vi "Check_Pos_L.vi"(0 "FPGA_Data":sgl[](array[numeric]), 2 "Q_MotorCmd_IN":refnum<queue>, 3 "Q_MotorCmd_Err_IN":errorcluster, 7 "Param_In":T1) -> (6 "LOAD_CELL_PEAK_L":sgl[](array[numeric]), 12 "Target_Pos":i32, 13 "Param_Out":T1, 14 "Flag":T2(ring), 15 "L_NUM":u32, 16 "Q_MotorCmd_OUT":refnum<queue>, 17 "Q_MotorCmd_Err_OUT":errorcluster, 18 "L_Period":u32, 19 "L_GCP":sgl)   [LabVIEW 2019]
uses:
  RT_GLOBAL.vi
panel:
  out "L_Period_EXT":u32
  out "L_GCP_EXT":sgl
  out "L_NUM_EXT":u32
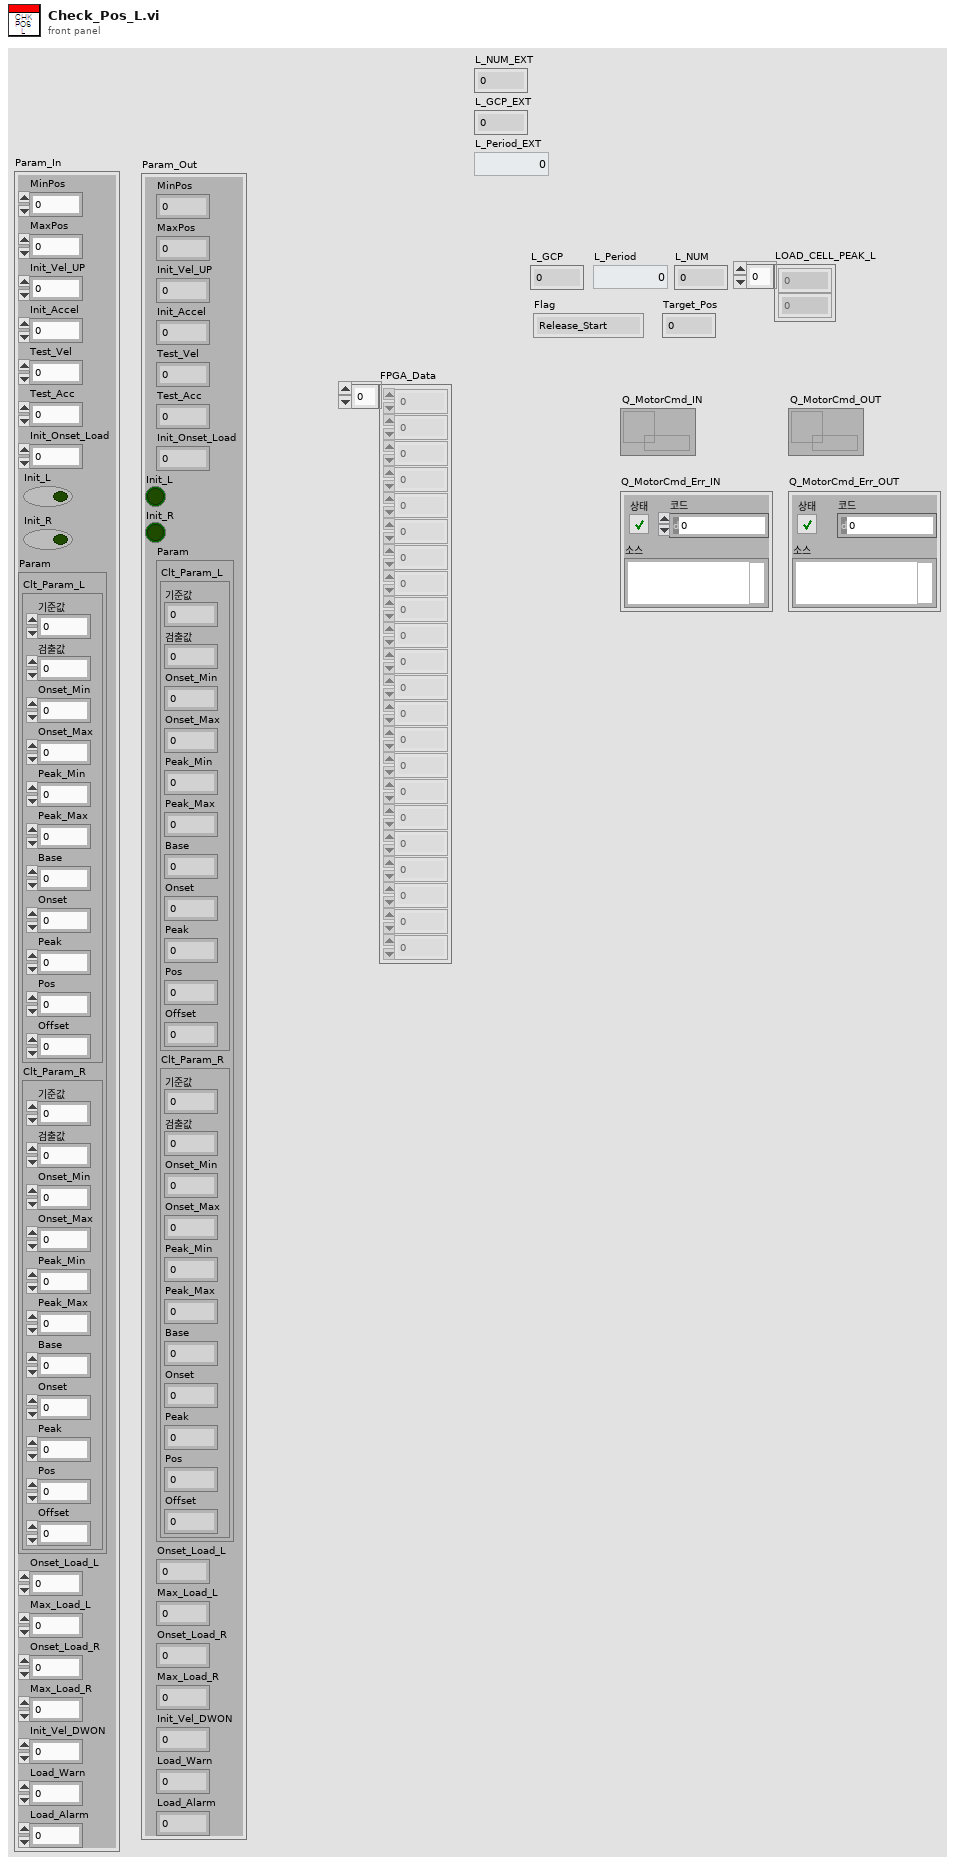
[diagram p1: front panel]
types:
  T1 = cluster{"MinPos":i32, "MaxPos":i32, "Init_Vel_UP":i32, "Init_Accel":u32, "Test_Vel":i32, "Test_Acc":u32, "Init_Onset_Load":sgl, "Init_L":bool, "Init_R":bool, "Param":cluster{"Clt_Param_L":cluster{"기준값":sgl, "검출값":sgl, "Onset_Min":sgl, "Onset_Max":sgl, "Peak_Min":sgl, "Peak_Max":sgl, "Base":i32, "Onset":i32, "Peak":i32, "Pos":i32, "Offset":sgl}, "Clt_Param_R":cluster{"기준값":sgl, "검출값":sgl, "Onset_Min":sgl, "Onset_Max":sgl, "Peak_Min":sgl, "Peak_Max":sgl, "Base":i32, "Onset":i32, "Peak":i32, "Pos":i32, "Offset":sgl}}, "Onset_Load_L":sgl, "Max_Load_L":sgl, "Onset_Load_R":sgl, "Max_Load_R":sgl, "Init_Vel_DWON":i32, "Load_Warn":sgl, "Load_Alarm":sgl}
  T2 = enum16{"Release_Start", "Onset_Start", "Peak_Start", "Calculate"}
  T3 = cluster{"Cmd":string, "Data1":variant, "Data2":variant}
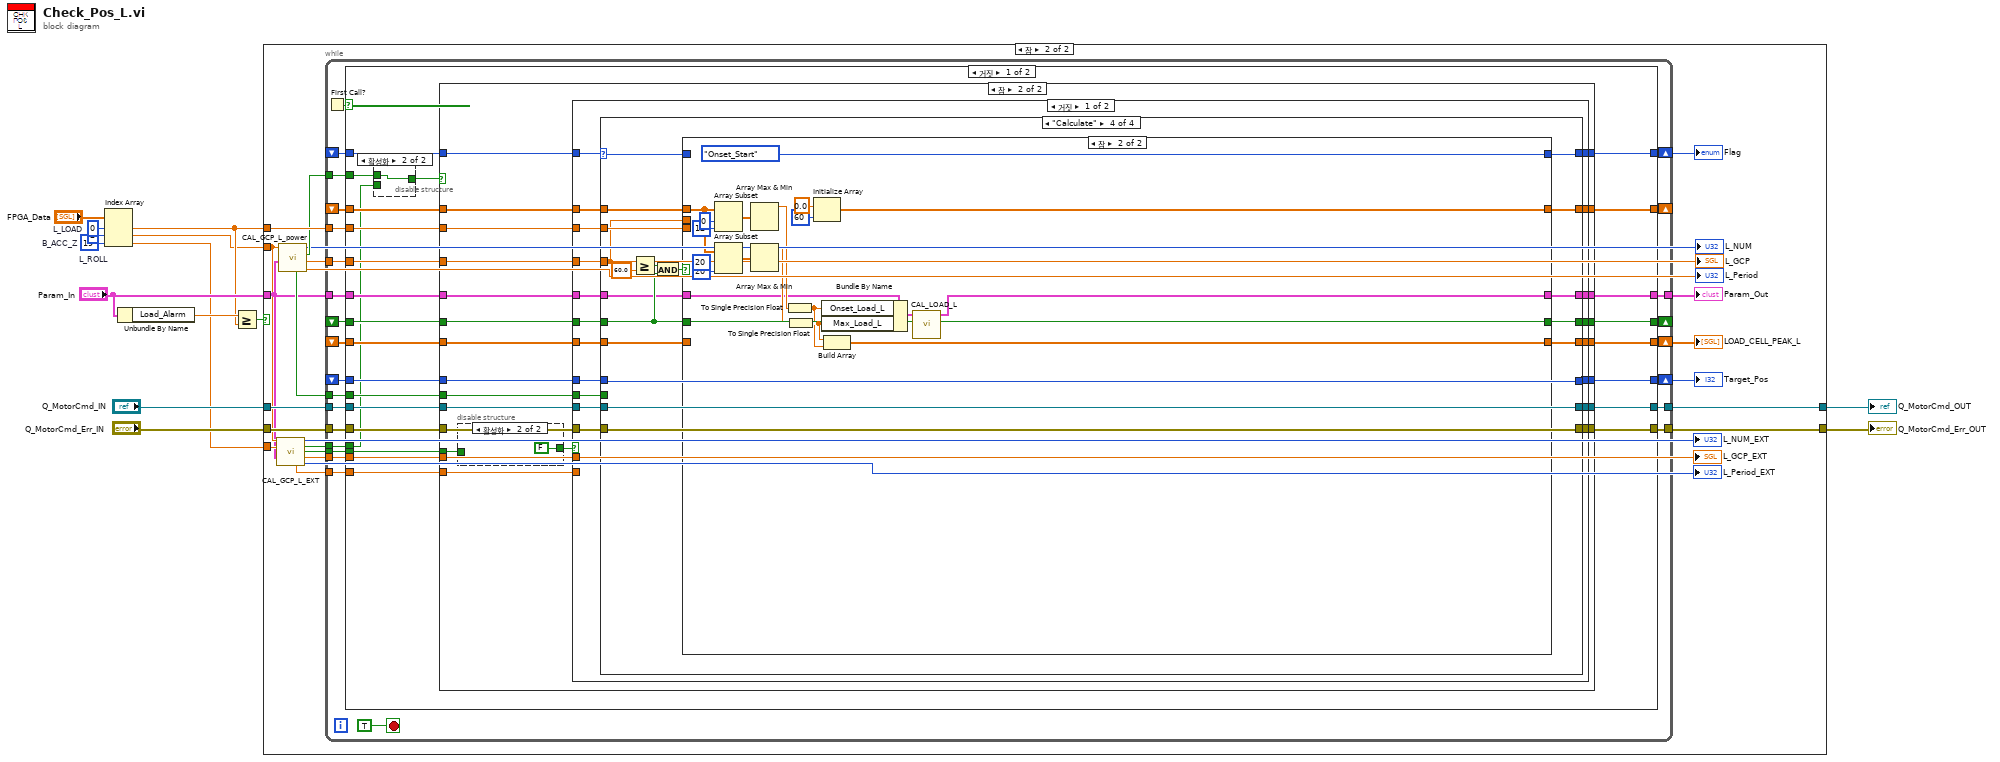
[diagram p0: block diagram]
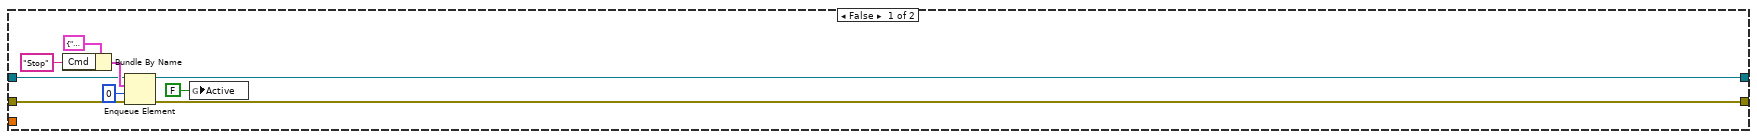
[diagram p2: hidden frame]
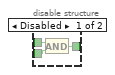
[diagram p3: hidden frame]
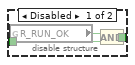
[diagram p5: hidden frame]
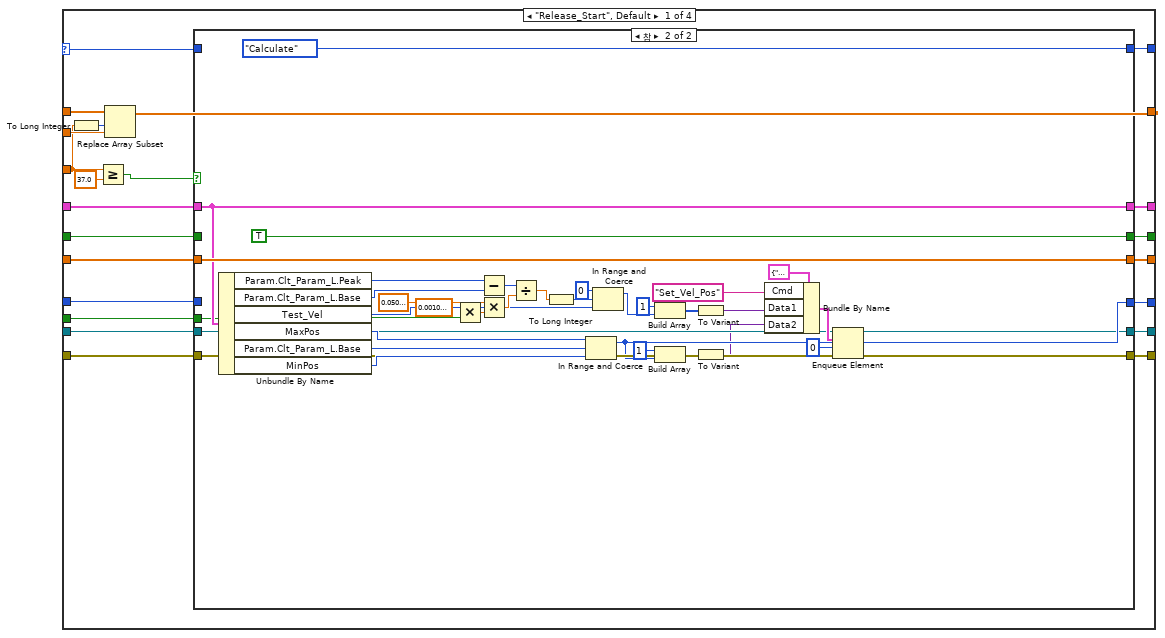
[diagram p6: hidden frame]
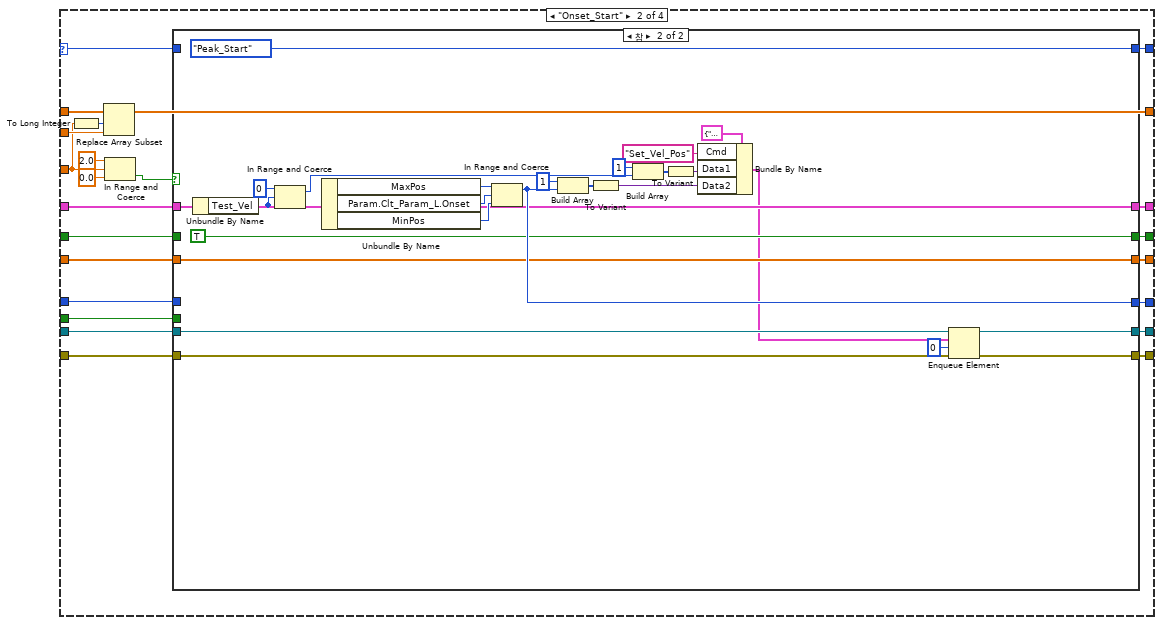
[diagram p8: hidden frame]
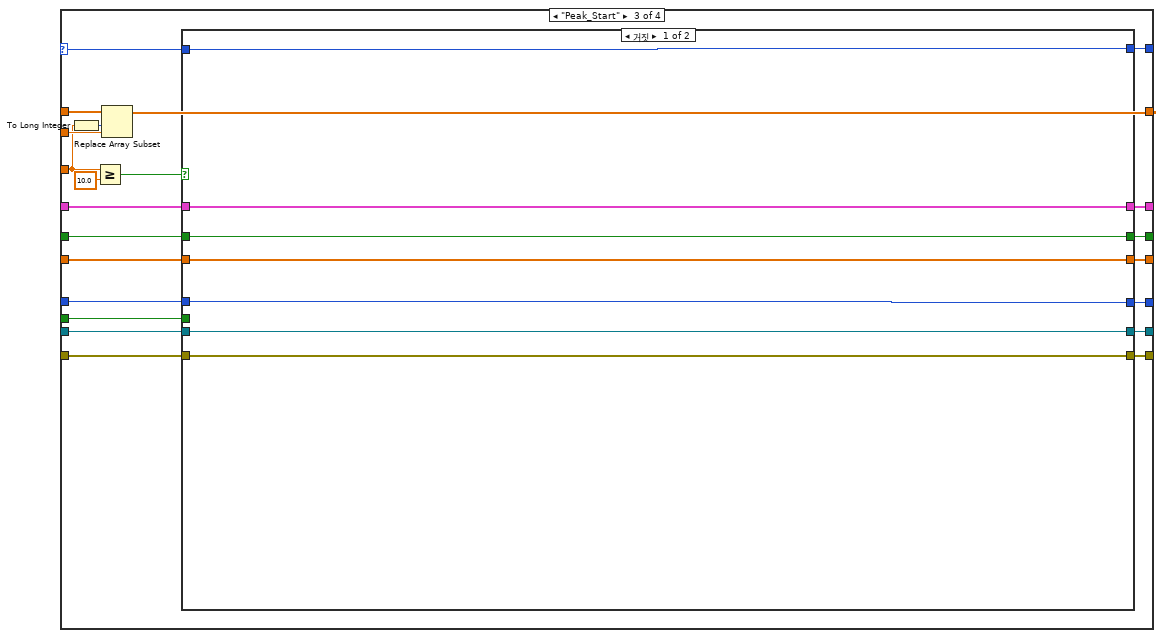
[diagram p10: hidden frame]
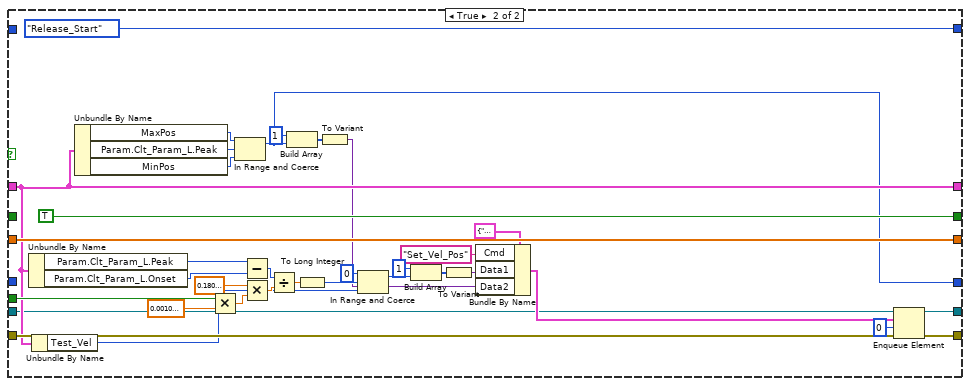
[diagram p11: hidden frame]
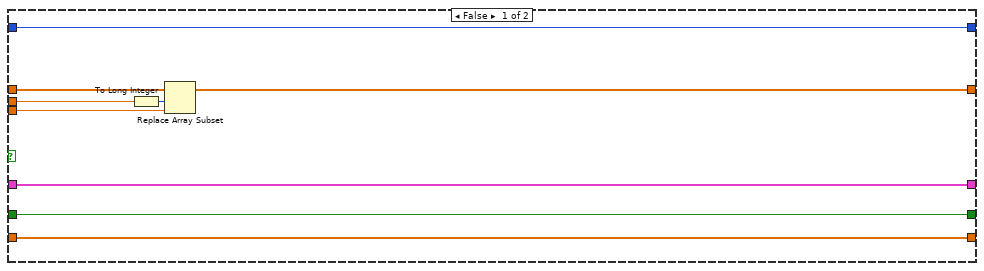
[diagram p12: hidden frame]
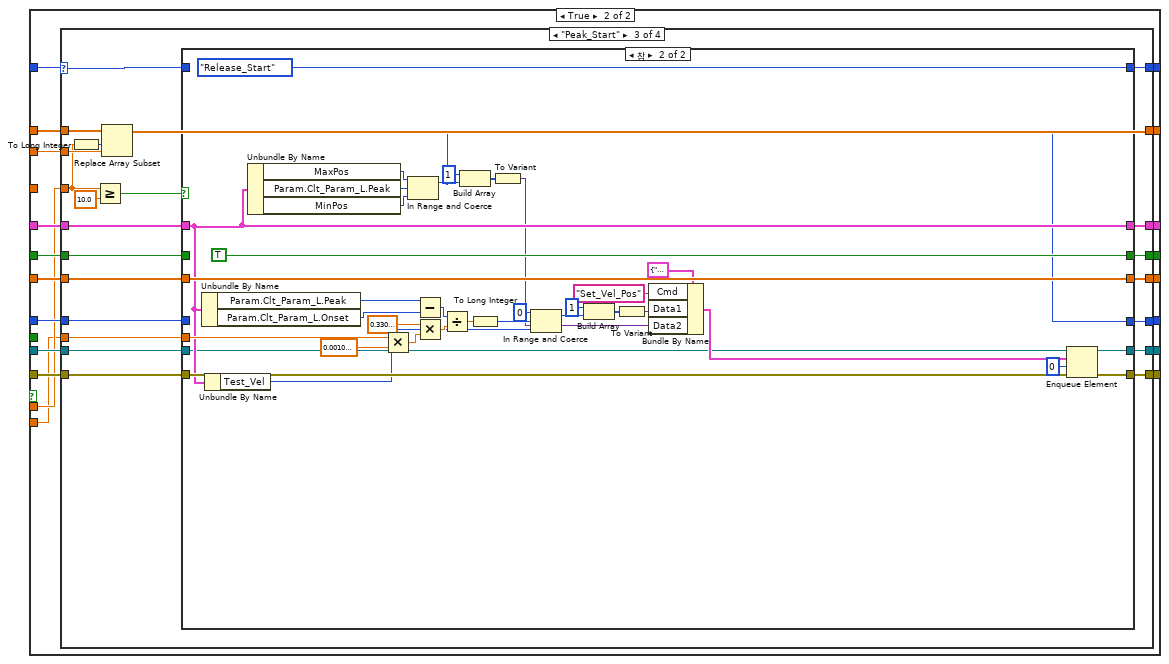
[diagram p13: hidden frame]
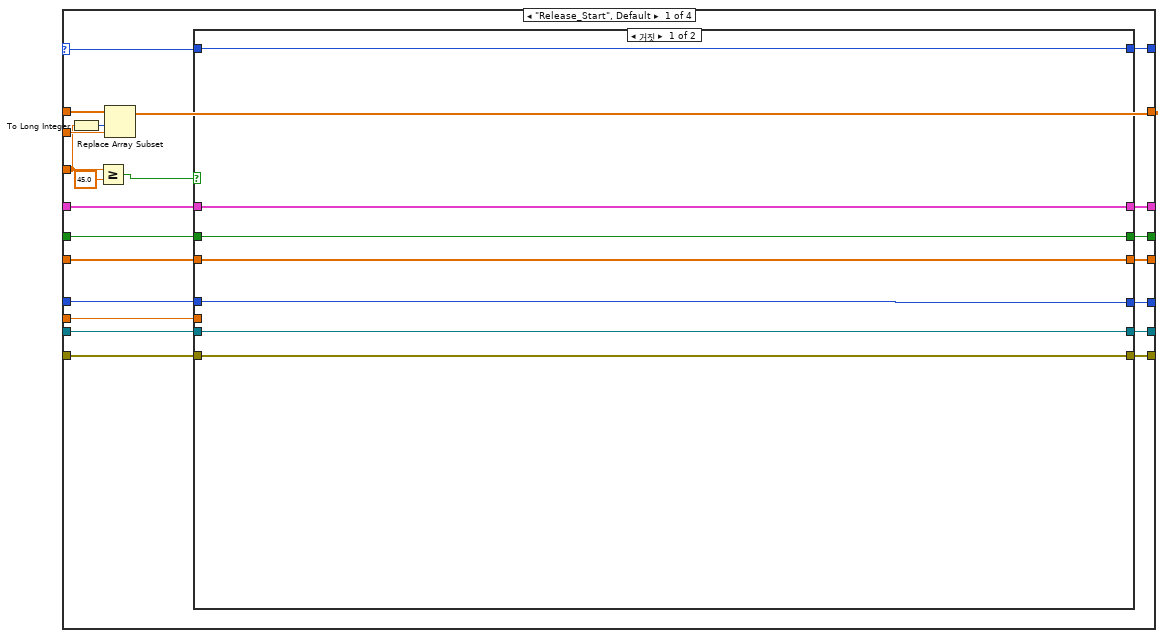
[diagram p14: hidden frame]
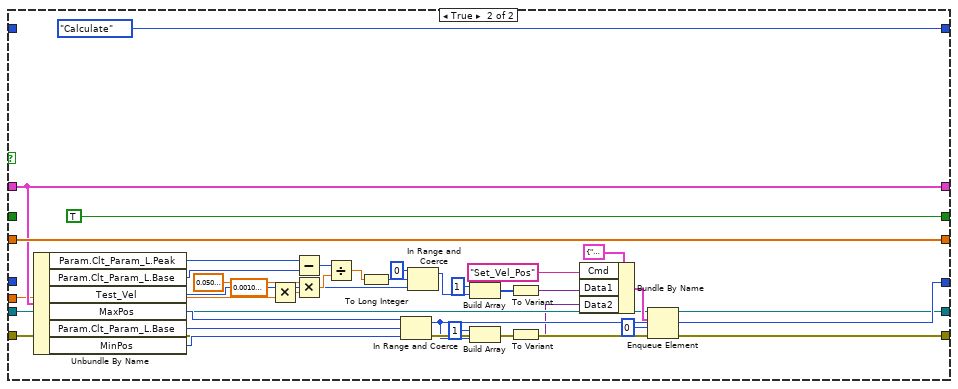
[diagram p15: hidden frame]
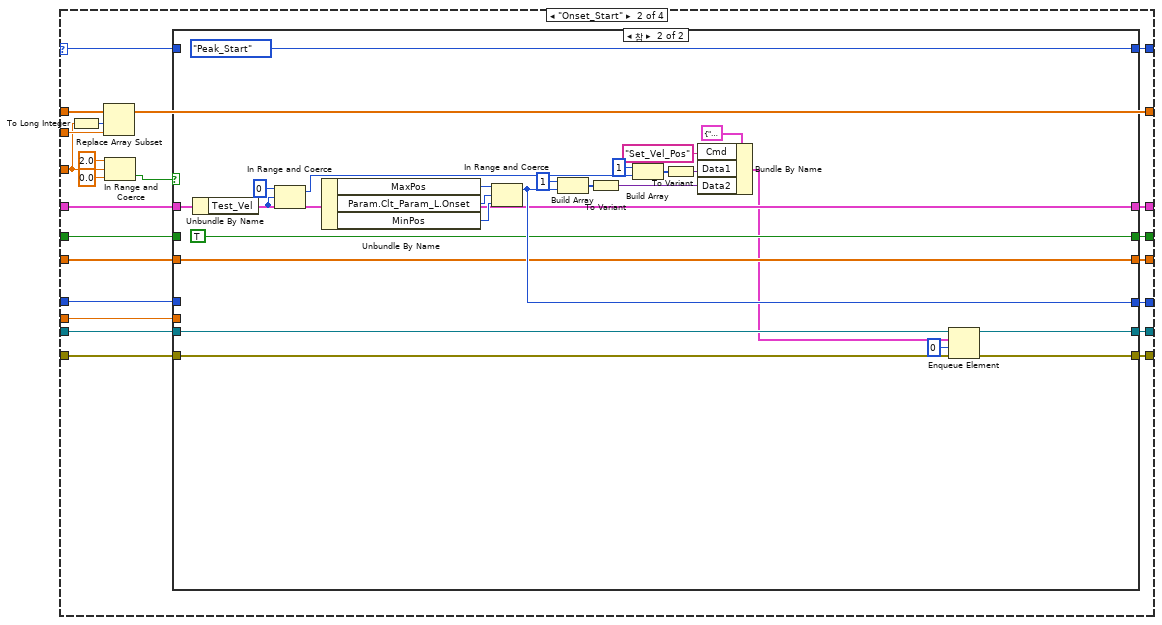
[diagram p16: hidden frame]
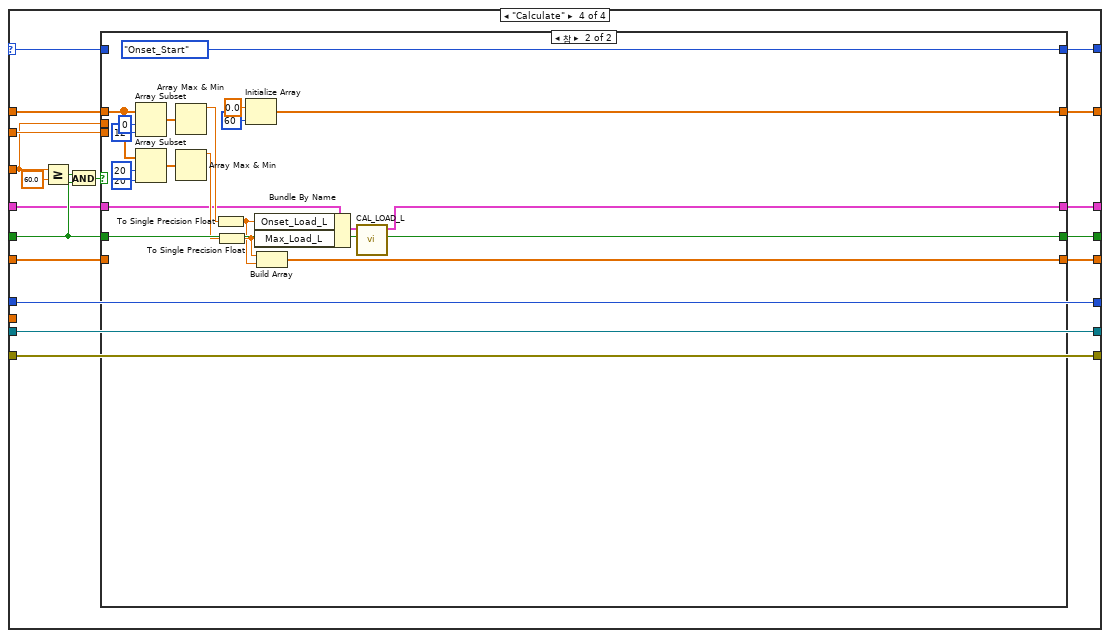
[diagram p19: hidden frame]
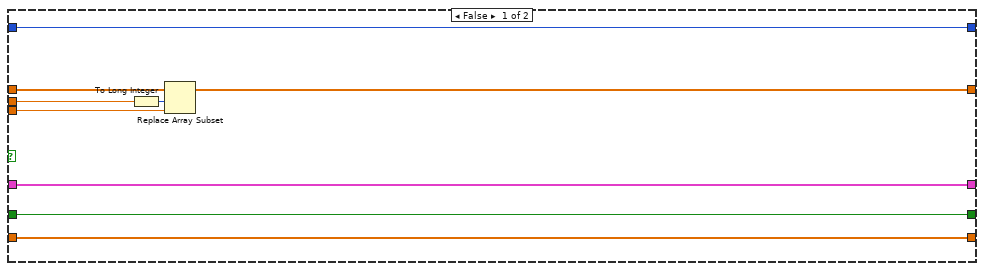
[diagram p20: hidden frame]
diagram:
  w4 = 19  # B_ACC_Z
  w6 = 2  # L_ROLL
  w8 = 0  # L_LOAD
  n1 = Index Array(array="FPGA_Data", index #1=w8, index #2=w6, index #3=w4) -> (element #1=w7:sgl, element #2=w5:sgl, element #3=w3:sgl)
  n2 = Unbundle By Name("Param_In") -> ("Load_Alarm"=w12:sgl)
  n3 = Greater Or Equal?(x=w12, y=w7) -> (x >= y?=w11:bool)
  n4 = case shown="참" w11 {
    tunnel: w5 -> [_ w34]
    tunnel: "Q_MotorCmd_IN" -> [w20 w46]
    tunnel: "Q_MotorCmd_Err_IN" -> [w19 w45]
    tunnel: "Param_In" -> [_ w32]
    tunnel: w7 -> [_ w44]
    tunnel: w3 -> [_ w33]
    tunnel: [w16 w25] -> w2
    tunnel: [w15 w24] -> w1
    frame False {
      n5 = Bundle By Name(cluster=T3 {"Cmd"="", "Data1"=variant, "Data2"=variant}, "Cmd"="Stop") -> (w21:T3)
      n6 = Enqueue Element(queue=w20, element=w21, timeout in ms (-1)=0 ("타임아웃(ms) (-1)"), error in (no error)=w19) -> (queue out=w16:refnum<queue>, error out=w15:errorcluster)  [unwired: 1 out]
      n7 = global write "RT_GLOBAL.vi" "Active"(FALSE ("Active")) -> ()
    }
    frame True {
      n8 = call "CAL_GCP_L_EXT.vi"("L_ROLL"=w34, "ACC_Z"=w33, "Param_In"=w32) -> ("L_NUM"=→"L_NUM_EXT":u32, "L_Ctrl_Start"=w29:bool, "L_RUN_OK"=w28:bool, "L_GCP_EXT"=w27:sgl, "L_GCP_Total_TIME"=w26:sgl, "L_Period"=→"L_Period_EXT":u32)  [unwired: 7 in]
      "L_GCP_EXT" <- w27
      n9 = call "CAL_GCP_L_power.vi"("출력 클러스터 2"=w32, "L_ROLL"=w34) -> ("L_Period"=→"L_Period":sgl, "L_GCP"=w42:sgl, "L_Ctrl_Start"=w43:bool, "L_NUM"=→"L_NUM":u32, "L_Run_OK"=w35:bool)  [unwired: 5 in]
      "L_GCP" <- w42
      n10 = while {
        tunnel: w43 -> [w70]
        tunnel: w42 -> [w56]
        shift-right: [w71] -> w39
        shift-left: _ -> [w62]
        shift-right: [w69] -> _
        shift-left: _ -> [w61]
        tunnel: w32 -> [w68]
        tunnel: [w67] -> w36
        shift-right: [w65] -> _
        shift-left: _ -> [w66]
        shift-right: [w64] -> w38
        shift-left: _ -> [w59]
        tunnel: w46 -> [w58]
        tunnel: w45 -> [w57]
        tunnel: w44 -> [w60]
        shift-right: [w55] -> w37
        shift-left: _ -> [w54]
        tunnel: w35 -> [w53]
        tunnel: w29 -> [w52]
        tunnel: w28 -> [w51]
        tunnel: w27 -> [w50]
        tunnel: w26 -> [w49]
        tunnel: [w48] -> w25
        tunnel: [w47] -> w24
        stop <- TRUE stop-if-true
        n11 = First Call?() -> (First Call?: T/F=w72:bool)
        n12 = case shown="거짓" w72 {
          tunnel: [w97 T2."Release_Start"] -> w71
          tunnel: w70 -> [w80 _]
          tunnel: [w94 w642] -> w69
          tunnel: [w91 w641] -> w67
          tunnel: w68 -> [w92 w641]
          tunnel: w66 -> [w89 _]
          tunnel: [w90 TRUE] -> w65
          tunnel: [w87 0] -> w64
          tunnel: w62 -> [w96 _]
          tunnel: w61 -> [w95 _]
          tunnel: w60 -> [w93 _]
          tunnel: w59 -> [w88 _]
          tunnel: w58 -> [w86 w636]
          tunnel: w57 -> [w85 w635]
          tunnel: w56 -> [w84 _]
          tunnel: [w83 w637] -> w55
          tunnel: w54 -> [w82 _]
          tunnel: w53 -> [w81 _]
          tunnel: w52 -> [w79 _]
          tunnel: w51 -> [w77 _]
          tunnel: w50 -> [w76 _]
          tunnel: w49 -> [w75 _]
          tunnel: [w74 w636] -> w48
          tunnel: [w73 w635] -> w47
          frame False {
            n13 = disable-structure shown="활성화" {
              disable-tunnel: w80 -> [w100 w101]
              disable-tunnel: w79 -> [w99 _]
              disable-tunnel: [w98 w101] -> w78
              frame Disabled {
                n14 = And(x=w100, y=w99) -> (x .and. y?=w98:bool)
              }
              frame Enabled {
              }
            }
            n15 = case shown="참" w78 {
              tunnel: [w109 w131] -> w97
              tunnel: w96 -> [w109 w132]
              tunnel: [w108 w129] -> w94
              tunnel: w95 -> [w108 w130]
              tunnel: w93 -> [_ w127]
              tunnel: [w107 w125] -> w91
              tunnel: w92 -> [w107 w126]
              tunnel: [w106 w124] -> w90
              tunnel: w89 -> [w106 w123]
              tunnel: [w105 w122] -> w87
              tunnel: w88 -> [w105 w121]
              tunnel: w86 -> [w103 w120]
              tunnel: w85 -> [w102 w119]
              tunnel: w84 -> [_ w128]
              tunnel: [w104 w118] -> w83
              tunnel: w82 -> [w104 w117]
              tunnel: w81 -> [_ w116]
              tunnel: w77 -> [_ w113]
              tunnel: w76 -> [_ w114]
              tunnel: w75 -> [_ w112]
              tunnel: [w103 w111] -> w74
              tunnel: [w102 w110] -> w73
              frame False {
              }
              frame True {
                n16 = disable-structure shown="활성화" {
                  disable-tunnel: [w135 FALSE] -> w115
                  disable-tunnel: w113 -> [w134 _]
                  frame Disabled {
                    n17 = global read "RT_GLOBAL.vi" "R_RUN_OK"() -> (w133:bool)
                    n18 = And(x=w133, y=w134) -> (x .and. y?=w135:bool)
                  }
                  frame Enabled {
                  }
                }
                n19 = case shown="거짓" w115 {
                  tunnel: w132 -> [w155 w404]
                  tunnel: [w154 w403] -> w131
                  tunnel: w130 -> [w153 w402]
                  tunnel: [w152 w401] -> w129
                  tunnel: w128 -> [w151 _]
                  tunnel: w127 -> [w150 w400]
                  tunnel: w126 -> [w149 w399]
                  tunnel: [w148 w398] -> w125
                  tunnel: [w147 w397] -> w124
                  tunnel: w123 -> [w146 w396]
                  tunnel: [w145 w395] -> w122
                  tunnel: w121 -> [w144 w394]
                  tunnel: w120 -> [w143 w393]
                  tunnel: w119 -> [w142 w392]
                  tunnel: [w141 w391] -> w118
                  tunnel: w117 -> [w140 w390]
                  tunnel: w116 -> [w139 _]
                  tunnel: w114 -> [_ w389]
                  tunnel: w112 -> [_ w388]
                  tunnel: [w138 w387] -> w111
                  tunnel: [w137 w386] -> w110
                  frame False {
                    n20 = case shown="\"Calculate\"" w155 {
                      selector: w155 -> [w175 w242 w296 w356]
                      tunnel: [w165 w241 w281 w355] -> w154
                      tunnel: w153 -> [w174 w237 w286 w354]
                      tunnel: [w166 w236 w285 w353] -> w152
                      tunnel: w151 -> [w167 w234 w282 w350]
                      tunnel: w150 -> [w173 w235 w283 w352]
                      tunnel: w149 -> [w172 w233 w295 w345]
                      tunnel: [w164 w232 w294 w344] -> w148
                      tunnel: [w163 w231 w293 w348] -> w147
                      tunnel: w146 -> [w171 w230 w288 w347]
                      tunnel: [w162 w229 w292 w341] -> w145
                      tunnel: w144 -> [w170 w228 w289 w341]
                      tunnel: w143 -> [w169 w227 w291 w340]
                      tunnel: w142 -> [w168 w226 w290 w339]
                      tunnel: [w160 w224 w279 w343] -> w141
                      tunnel: w140 -> [w161 w225 w280 w342]
                      tunnel: w139 -> [w159 w223 w278 _]
                      tunnel: [w157 w221 w276 w340] -> w138
                      tunnel: [w156 w220 w275 w339] -> w137
                      frame "Release_Start", Default {
                        n21 = To Long Integer(number=w167) -> (32bit integer=w176:i32)
                        n22 = Greater Or Equal?(x=w167, y=sgl 37.0) -> (x >= y?=w158:bool)
                        n23 = Replace Array Subset(array=w174, new element=w173, index=w176) -> (w166:sgl[])
                        n24 = case shown="참" w158 {
                          tunnel: w175 -> [w184 _]
                          tunnel: [w184 T2."Calculate"] -> w165
                          tunnel: [w183 w202] -> w164
                          tunnel: w172 -> [w183 w202]
                          tunnel: [w182 TRUE] -> w163
                          tunnel: w171 -> [w182 _]
                          tunnel: [w181 w188] -> w162
                          tunnel: w170 -> [w181 _]
                          tunnel: w169 -> [w179 w203]
                          tunnel: w168 -> [w178 w204]
                          tunnel: w161 -> [w180 w214]
                          tunnel: [w180 w214] -> w160
                          tunnel: w159 -> [_ w192]
                          tunnel: [w179 w186] -> w157
                          tunnel: [w178 w185] -> w156
                          frame False {
                          }
                          frame True {
                            n25 = Unbundle By Name(w202) -> ("Param.Clt_Param_L.Peak"=w196:i32, "Param.Clt_Param_L.Base"=w195:i32, "Test_Vel"=w197:i32, "MaxPos"=w217:i32, "Param.Clt_Param_L.Base"=w218:i32, "MinPos"=w216:i32)
                            n26 = Multiply(x=sgl 0.001 ("y"), y=w192) -> (x*y=w194:sgl)
                            n27 = Subtract(x=w196, y=w195) -> (x-y=w209:i32)
                            n28 = Multiply(x=sgl 0.05 ("y"), y=w194) -> (x*y=w213:sgl)
                            n29 = Divide(x=w209, y=w213) -> (x/y=w208:sgl)
                            n30 = To Long Integer(number=w208) -> (32bit integer=w199:i32)
                            n31 = In Range and Coerce(upper limit=w217, x=w218, lower limit=w216) -> (coerced(x)=w188:i32)  [unwired: 1 out]
                            n32 = In Range and Coerce(upper limit=0, x=w199, lower limit=w197) -> (coerced(x)=w201:i32)  [unwired: 1 out]
                            n33 = Build Array(1 ("원소"), w201) -> (w210:i32[])
                            n34 = Build Array(1 ("원소"), w188) -> (w190:i32[])
                            n35 = To Variant(anything=w210) -> (Variant=w211:variant)
                            n36 = To Variant(anything=w190) -> (Variant=w187:variant)
                            n37 = Bundle By Name(cluster=T3 {"Cmd"="", "Data1"=variant, "Data2"=variant}, "Cmd"="Set_Vel_Pos", "Data1"=w211, "Data2"=w187) -> (w212:T3)
                            n38 = Enqueue Element(queue=w203, element=w212, timeout in ms (-1)=0 ("타임아웃(ms) (-1)"), error in (no error)=w204) -> (queue out=w186:refnum<queue>, error out=w185:errorcluster)  [unwired: 1 out]
                          }
                        }
                      }
                      frame "Onset_Start" {
                        n39 = To Long Integer(number=w234) -> (32bit integer=w238:i32)
                        n40 = Replace Array Subset(array=w237, new element=w235, index=w238) -> (w236:sgl[])
                        n41 = In Range and Coerce(upper limit=sgl 2.0 ("상위 리미트"), x=w234, lower limit=sgl 0.0 ("하위 리미트")) -> (In Range?=w222:bool)  [unwired: 1 out]
                        n42 = case shown="참" w222 {
                          tunnel: w242 -> [w249 _]
                          tunnel: [w249 T2."Peak_Start"] -> w241
                          tunnel: [w248 w256] -> w232
                          tunnel: w233 -> [w248 w256]
                          tunnel: [w247 TRUE] -> w231
                          tunnel: w230 -> [w247 _]
                          tunnel: [w246 w268] -> w229
                          tunnel: w228 -> [w246 _]
                          tunnel: w227 -> [w244 w260]
                          tunnel: w226 -> [w243 w259]
                          tunnel: w225 -> [w245 w266]
                          tunnel: [w245 w266] -> w224
                          tunnel: w223 -> [_ _]
                          tunnel: [w244 w251] -> w221
                          tunnel: [w243 w250] -> w220
                          frame False {
                          }
                          frame True {
                            n43 = Unbundle By Name(w256) -> ("Test_Vel"=w255:i32)
                            n44 = In Range and Coerce(upper limit=0, x=w255, lower limit=w255) -> (coerced(x)=w257:i32)  [unwired: 1 out]
                            n45 = Unbundle By Name(w256) -> ("MaxPos"=w270:i32, "Param.Clt_Param_L.Onset"=w271:i32, "MinPos"=w269:i32)
                            n46 = In Range and Coerce(upper limit=w270, x=w271, lower limit=w269) -> (coerced(x)=w268:i32)  [unwired: 1 out]
                            n47 = Build Array(1 ("원소"), w268) -> (w273:i32[])
                            n48 = To Variant(anything=w273) -> (Variant=w252:variant)
                            n49 = Build Array(1 ("원소"), w257) -> (w265:i32[])
                            n50 = To Variant(anything=w265) -> (Variant=w264:variant)
                            n51 = Bundle By Name(cluster=T3 {"Cmd"="", "Data1"=variant, "Data2"=variant}, "Cmd"="Set_Vel_Pos", "Data1"=w264, "Data2"=w252) -> (w254:T3)
                            n52 = Enqueue Element(queue=w260, element=w254, timeout in ms (-1)=0 ("타임아웃(ms) (-1)"), error in (no error)=w259) -> (queue out=w251:refnum<queue>, error out=w250:errorcluster)  [unwired: 1 out]
                          }
                        }
                      }
                      frame "Peak_Start" {
                        n53 = To Long Integer(number=w282) -> (32bit integer=w284:i32)
                        n54 = Greater Or Equal?(x=w282, y=sgl 10.0) -> (x >= y?=w277:bool)
                        n55 = Replace Array Subset(array=w286, new element=w283, index=w284) -> (w285:sgl[])
                        n56 = case shown="거짓" w277 {
                          tunnel: w296 -> [w303 _]
                          tunnel: [w303 T2."Release_Start"] -> w281
                          tunnel: [w302 w315] -> w294
                          tunnel: w295 -> [w302 w315]
                          tunnel: [w301 TRUE] -> w293
                          tunnel: w288 -> [w301 _]
                          tunnel: [w300 w306] -> w292
                          tunnel: w289 -> [w300 _]
                          tunnel: w291 -> [w298 w307]
                          tunnel: w290 -> [w297 w319]
                          tunnel: w280 -> [w299 w331]
                          tunnel: [w299 w331] -> w279
                          tunnel: w278 -> [_ w318]
                          tunnel: [w298 w305] -> w276
                          tunnel: [w297 w304] -> w275
                          frame False {
                          }
                          frame True {
                            n57 = Unbundle By Name(w315) -> ("Param.Clt_Param_L.Peak"=w327:i32, "Param.Clt_Param_L.Onset"=w326:i32)
                            n58 = Unbundle By Name(w315) -> ("Test_Vel"=w314:i32)
                            n59 = Unbundle By Name(w315) -> ("MaxPos"=w334:i32, "Param.Clt_Param_L.Peak"=w335:i32, "MinPos"=w333:i32)
                            n60 = Multiply(x=w318, y=sgl 0.001) -> (x*y=w311:sgl)
                            n61 = In Range and Coerce(upper limit=w334, x=w335, lower limit=w333) -> (coerced(x)=w306:i32)  [unwired: 1 out]
                            n62 = Subtract(x=w327, y=w326) -> (x-y=w325:i32)
                            n63 = Multiply(x=sgl 0.18 ("y"), y=w311) -> (x*y=w330:sgl)
                            n64 = Divide(x=w325, y=w330) -> (x/y=w324:sgl)
                            n65 = Build Array(1 ("원소"), w306) -> (w337:i32[])
                            n66 = To Long Integer(number=w324) -> (32bit integer=w313:i32)
                            n67 = To Variant(anything=w337) -> (Variant=w308:variant)
                            n68 = In Range and Coerce(upper limit=0, x=w313, lower limit=w314) -> (coerced(x)=w316:i32)  [unwired: 1 out]
                            n69 = Build Array(u32 1 ("원소"), w316) -> (w328:u32[])
                            n70 = To Variant(anything=w328) -> (Variant=w329:variant)
                            n71 = Bundle By Name(cluster=T3 {"Cmd"="", "Data1"=variant, "Data2"=variant}, "Cmd"="Set_Vel_Pos", "Data1"=w329, "Data2"=w308) -> (w309:T3)
                            n72 = Enqueue Element(queue=w307, element=w309, timeout in ms (-1)=0 ("타임아웃(ms) (-1)"), error in (no error)=w319) -> (queue out=w305:refnum<queue>, error out=w304:errorcluster)  [unwired: 1 out]
                          }
                        }
                      }
                      frame "Calculate" {
                        n73 = Greater Or Equal?(x=w350, y=sgl 60.0) -> (x >= y?=w349:bool)
                        n74 = And(x=w349, y=w347) -> (x .and. y?=w346:bool)
                        n75 = case shown="참" w346 {
                          tunnel: [w365 T2."Onset_Start"] -> w355
                          tunnel: w356 -> [w365 _]
                          tunnel: w354 -> [w363 w378]
                          tunnel: [w362 w382] -> w353
                          tunnel: w350 -> [w361 _]
                          tunnel: w352 -> [w360 _]
                          tunnel: [w359 w381] -> w348
                          tunnel: w347 -> [w359 w381]
                          tunnel: w345 -> [w358 w367]
                          tunnel: [w358 w379] -> w344
                          tunnel: [w357 w366] -> w343
                          tunnel: w342 -> [w357 _]
                          frame False {
                            n76 = To Long Integer(number=w361) -> (32bit integer=w364:i32)
                            n77 = Replace Array Subset(array=w363, new element=w360, index=w364) -> (w362:sgl[])
                          }
                          frame True {
                            n78 = Array Subset(array=w378, index=0 ("인덱스"), length=12 ("길이")) -> (w377:sgl[])
                            n79 = Array Subset(array=w378, index=20 ("인덱스"), length=20 ("길이")) -> (w376:sgl[])
                            n80 = Array Max & Min(array=w377) -> (max value=w371:sgl)  [unwired: 3 out]
                            n81 = Array Max & Min(array=w376) -> (max value=w370:sgl)  [unwired: 3 out]
                            n82 = To Single Precision Float(number=w371) -> (single precision float=w368:sgl)
                            n83 = To Single Precision Float(number=w370) -> (single precision float=w369:sgl)
                            n84 = Initialize Array(sgl 0.0 ("원소"), 60 ("차원 크기")) -> (w382:sgl[])
                            n85 = Bundle By Name(cluster=w367, "Onset_Load_L"=w368, "Max_Load_L"=w369) -> (w380:T1)
                            n86 = Build Array(w369, w368) -> (w366:sgl[])
                            n87 = call "CAL_LOAD_L.vi"("Param_In"=w380) -> ("Param_Out"=w379:T1)  [unwired: 10 in]
                          }
                        }
                      }
                    }
                  }
                  frame True {
                    n88 = case shown="\"Peak_Start\"" w404 {
                      selector: w404 -> [w424 w491 w545 w605]
                      tunnel: [w414 w490 w530 w604] -> w403
                      tunnel: w402 -> [w423 w486 w535 w603]
                      tunnel: [w415 w485 w534 w602] -> w401
                      tunnel: w389 -> [w416 w483 w531 w599]
                      tunnel: w400 -> [w422 w484 w532 w601]
                      tunnel: w399 -> [w421 w482 w544 w594]
                      tunnel: [w413 w481 w543 w593] -> w398
                      tunnel: [w412 w480 w542 w597] -> w397
                      tunnel: w396 -> [w420 w479 w537 w596]
                      tunnel: [w411 w478 w541 w590] -> w395
                      tunnel: w394 -> [w419 w477 w538 w590]
                      tunnel: w393 -> [w418 w476 w540 w589]
                      tunnel: w392 -> [w417 w475 w539 w588]
                      tunnel: [w409 w473 w528 w592] -> w391
                      tunnel: w390 -> [w410 w474 w529 w591]
                      tunnel: w388 -> [w408 w472 w527 _]
                      tunnel: [w406 w470 w525 w589] -> w387
                      tunnel: [w405 w469 w524 w588] -> w386
                      frame "Release_Start", Default {
                        n89 = To Long Integer(number=w416) -> (32bit integer=w425:i32)
                        n90 = Greater Or Equal?(x=w416, y=sgl 45.0) -> (x >= y?=w407:bool)
                        n91 = Replace Array Subset(array=w423, new element=w422, index=w425) -> (w415:sgl[])
                        n92 = case shown="거짓" w407 {
                          tunnel: w424 -> [w433 _]
                          tunnel: [w433 T2."Calculate"] -> w414
                          tunnel: [w432 w451] -> w413
                          tunnel: w421 -> [w432 w451]
                          tunnel: [w431 TRUE] -> w412
                          tunnel: w420 -> [w431 _]
                          tunnel: [w430 w437] -> w411
                          tunnel: w419 -> [w430 _]
                          tunnel: w418 -> [w428 w452]
                          tunnel: w417 -> [w427 w453]
                          tunnel: w410 -> [w429 w463]
                          tunnel: [w429 w463] -> w409
                          tunnel: w408 -> [_ w441]
                          tunnel: [w428 w435] -> w406
                          tunnel: [w427 w434] -> w405
                          frame False {
                          }
                          frame True {
                            n93 = Unbundle By Name(w451) -> ("Param.Clt_Param_L.Peak"=w445:i32, "Param.Clt_Param_L.Base"=w444:i32, "Test_Vel"=w446:i32, "MaxPos"=w466:i32, "Param.Clt_Param_L.Base"=w467:i32, "MinPos"=w465:i32)
                            n94 = Multiply(x=sgl 0.001 ("y"), y=w441) -> (x*y=w443:sgl)
                            n95 = Subtract(x=w445, y=w444) -> (x-y=w458:i32)
                            n96 = Multiply(x=sgl 0.05 ("y"), y=w443) -> (x*y=w462:sgl)
                            n97 = Divide(x=w458, y=w462) -> (x/y=w457:sgl)
                            n98 = To Long Integer(number=w457) -> (32bit integer=w448:i32)
                            n99 = In Range and Coerce(upper limit=w466, x=w467, lower limit=w465) -> (coerced(x)=w437:i32)  [unwired: 1 out]
                            n100 = In Range and Coerce(upper limit=0, x=w448, lower limit=w446) -> (coerced(x)=w450:i32)  [unwired: 1 out]
                            n101 = Build Array(1 ("원소"), w450) -> (w459:i32[])
                            n102 = Build Array(1 ("원소"), w437) -> (w439:i32[])
                            n103 = To Variant(anything=w459) -> (Variant=w460:variant)
                            n104 = To Variant(anything=w439) -> (Variant=w436:variant)
                            n105 = Bundle By Name(cluster=T3 {"Cmd"="", "Data1"=variant, "Data2"=variant}, "Cmd"="Set_Vel_Pos", "Data1"=w460, "Data2"=w436) -> (w461:T3)
                            n106 = Enqueue Element(queue=w452, element=w461, timeout in ms (-1)=0 ("타임아웃(ms) (-1)"), error in (no error)=w453) -> (queue out=w435:refnum<queue>, error out=w434:errorcluster)  [unwired: 1 out]
                          }
                        }
                      }
                      frame "Onset_Start" {
                        n107 = To Long Integer(number=w483) -> (32bit integer=w487:i32)
                        n108 = Replace Array Subset(array=w486, new element=w484, index=w487) -> (w485:sgl[])
                        n109 = In Range and Coerce(upper limit=sgl 2.0 ("상위 리미트"), x=w483, lower limit=sgl 0.0 ("하위 리미트")) -> (In Range?=w471:bool)  [unwired: 1 out]
                        n110 = case shown="참" w471 {
                          tunnel: w491 -> [w498 _]
                          tunnel: [w498 T2."Peak_Start"] -> w490
                          tunnel: [w497 w505] -> w481
                          tunnel: w482 -> [w497 w505]
                          tunnel: [w496 TRUE] -> w480
                          tunnel: w479 -> [w496 _]
                          tunnel: [w495 w517] -> w478
                          tunnel: w477 -> [w495 _]
                          tunnel: w476 -> [w493 w509]
                          tunnel: w475 -> [w492 w508]
                          tunnel: w474 -> [w494 w515]
                          tunnel: [w494 w515] -> w473
                          tunnel: w472 -> [_ _]
                          tunnel: [w493 w500] -> w470
                          tunnel: [w492 w499] -> w469
                          frame False {
                          }
                          frame True {
                            n111 = Unbundle By Name(w505) -> ("Test_Vel"=w504:i32)
                            n112 = In Range and Coerce(upper limit=0, x=w504, lower limit=w504) -> (coerced(x)=w506:i32)  [unwired: 1 out]
                            n113 = Unbundle By Name(w505) -> ("MaxPos"=w519:i32, "Param.Clt_Param_L.Onset"=w520:i32, "MinPos"=w518:i32)
                            n114 = In Range and Coerce(upper limit=w519, x=w520, lower limit=w518) -> (coerced(x)=w517:i32)  [unwired: 1 out]
                            n115 = Build Array(1 ("원소"), w517) -> (w522:i32[])
                            n116 = To Variant(anything=w522) -> (Variant=w501:variant)
                            n117 = Build Array(1 ("원소"), w506) -> (w514:i32[])
                            n118 = To Variant(anything=w514) -> (Variant=w513:variant)
                            n119 = Bundle By Name(cluster=T3 {"Cmd"="", "Data1"=variant, "Data2"=variant}, "Cmd"="Set_Vel_Pos", "Data1"=w513, "Data2"=w501) -> (w503:T3)
                            n120 = Enqueue Element(queue=w509, element=w503, timeout in ms (-1)=0 ("타임아웃(ms) (-1)"), error in (no error)=w508) -> (queue out=w500:refnum<queue>, error out=w499:errorcluster)  [unwired: 1 out]
                          }
                        }
                      }
                      frame "Peak_Start" {
                        n121 = To Long Integer(number=w531) -> (32bit integer=w533:i32)
                        n122 = Greater Or Equal?(x=w531, y=sgl 10.0) -> (x >= y?=w526:bool)
                        n123 = Replace Array Subset(array=w535, new element=w532, index=w533) -> (w534:sgl[])
                        n124 = case shown="참" w526 {
                          tunnel: w545 -> [w552 _]
                          tunnel: [w552 T2."Release_Start"] -> w530
                          tunnel: [w551 w564] -> w543
                          tunnel: w544 -> [w551 w564]
                          tunnel: [w550 TRUE] -> w542
                          tunnel: w537 -> [w550 _]
                          tunnel: [w549 w555] -> w541
                          tunnel: w538 -> [w549 _]
                          tunnel: w540 -> [w547 w556]
                          tunnel: w539 -> [w546 w568]
                          tunnel: w529 -> [w548 w580]
                          tunnel: [w548 w580] -> w528
                          tunnel: w527 -> [_ w567]
                          tunnel: [w547 w554] -> w525
                          tunnel: [w546 w553] -> w524
                          frame False {
                          }
                          frame True {
                            n125 = Unbundle By Name(w564) -> ("Param.Clt_Param_L.Peak"=w576:i32, "Param.Clt_Param_L.Onset"=w575:i32)
                            n126 = Unbundle By Name(w564) -> ("Test_Vel"=w563:i32)
                            n127 = Unbundle By Name(w564) -> ("MaxPos"=w583:i32, "Param.Clt_Param_L.Peak"=w584:i32, "MinPos"=w582:i32)
                            n128 = Multiply(x=w567, y=sgl 0.001) -> (x*y=w560:sgl)
                            n129 = In Range and Coerce(upper limit=w583, x=w584, lower limit=w582) -> (coerced(x)=w555:i32)  [unwired: 1 out]
                            n130 = Subtract(x=w576, y=w575) -> (x-y=w574:i32)
                            n131 = Multiply(x=sgl 0.33 ("y"), y=w560) -> (x*y=w579:sgl)
                            n132 = Divide(x=w574, y=w579) -> (x/y=w573:sgl)
                            n133 = Build Array(1 ("원소"), w555) -> (w586:i32[])
                            n134 = To Long Integer(number=w573) -> (32bit integer=w562:i32)
                            n135 = To Variant(anything=w586) -> (Variant=w557:variant)
                            n136 = In Range and Coerce(upper limit=0, x=w562, lower limit=w563) -> (coerced(x)=w565:i32)  [unwired: 1 out]
                            n137 = Build Array(1 ("원소"), w565) -> (w577:i32[])
                            n138 = To Variant(anything=w577) -> (Variant=w578:variant)
                            n139 = Bundle By Name(cluster=T3 {"Cmd"="", "Data1"=variant, "Data2"=variant}, "Cmd"="Set_Vel_Pos", "Data1"=w578, "Data2"=w557) -> (w558:T3)
                            n140 = Enqueue Element(queue=w556, element=w558, timeout in ms (-1)=0 ("타임아웃(ms) (-1)"), error in (no error)=w568) -> (queue out=w554:refnum<queue>, error out=w553:errorcluster)  [unwired: 1 out]
                          }
                        }
                      }
                      frame "Calculate" {
                        n141 = Greater Or Equal?(x=w599, y=sgl 60.0) -> (x >= y?=w598:bool)
                        n142 = And(x=w598, y=w596) -> (x .and. y?=w595:bool)
                        n143 = case shown="참" w595 {
                          tunnel: [w614 T2."Onset_Start"] -> w604
                          tunnel: w605 -> [w614 _]
                          tunnel: w603 -> [w612 w627]
                          tunnel: [w611 w631] -> w602
                          tunnel: w599 -> [w610 _]
                          tunnel: w601 -> [w609 _]
                          tunnel: [w608 w630] -> w597
                          tunnel: w596 -> [w608 w630]
                          tunnel: w594 -> [w607 w616]
                          tunnel: [w607 w628] -> w593
                          tunnel: [w606 w615] -> w592
                          tunnel: w591 -> [w606 _]
                          frame False {
                            n144 = To Long Integer(number=w610) -> (32bit integer=w613:i32)
                            n145 = Replace Array Subset(array=w612, new element=w609, index=w613) -> (w611:sgl[])
                          }
                          frame True {
                            n146 = Array Subset(array=w627, index=0 ("인덱스"), length=12 ("길이")) -> (w626:sgl[])
                            n147 = Array Subset(array=w627, index=20 ("인덱스"), length=20 ("길이")) -> (w625:sgl[])
                            n148 = Array Max & Min(array=w626) -> (max value=w620:sgl)  [unwired: 3 out]
                            n149 = Array Max & Min(array=w625) -> (max value=w619:sgl)  [unwired: 3 out]
                            n150 = To Single Precision Float(number=w620) -> (single precision float=w617:sgl)
                            n151 = To Single Precision Float(number=w619) -> (single precision float=w618:sgl)
                            n152 = Initialize Array(sgl 0.0 ("원소"), 60 ("차원 크기")) -> (w631:sgl[])
                            n153 = Bundle By Name(cluster=w616, "Onset_Load_L"=w617, "Max_Load_L"=w618) -> (w629:T1)
                            n154 = Build Array(w618, w617) -> (w615:sgl[])
                            n155 = call "CAL_LOAD_L.vi"("Param_In"=w629) -> ("Param_Out"=w628:T1)  [unwired: 10 in]
                          }
                        }
                      }
                    }
                  }
                }
              }
            }
          }
          frame True {
            w638 = sgl 0.0
            n156 = Build Array(w638, w638) -> (w637:sgl[])
            n157 = Initialize Array(sgl 0.0 ("원소"), 60 ("차원 크기")) -> (w642:sgl[])
          }
        }
      }
      "Flag" <- w39
      "Target_Pos" <- w38
      "LOAD_CELL_PEAK_L" <- w37
      "Param_Out" <- w36
    }
  }
  "Q_MotorCmd_Err_OUT" <- w1
  "Q_MotorCmd_OUT" <- w2
